vi "GetDough.vi"(8 "error in (no error)":errorcluster, 11 "object in":refnum<class "Pizza(Product).lvclass">) -> (0 "error out":errorcluster, 2 "Dough":string, 3 "object out":refnum<class "Pizza(Product).lvclass">)   [LabVIEW 2014, in "Pizza(Product).lvclass"]
uses:
  Pizza(Product).lvclass
  Pizza(Product).lvclass/Pizza(Product).ctl
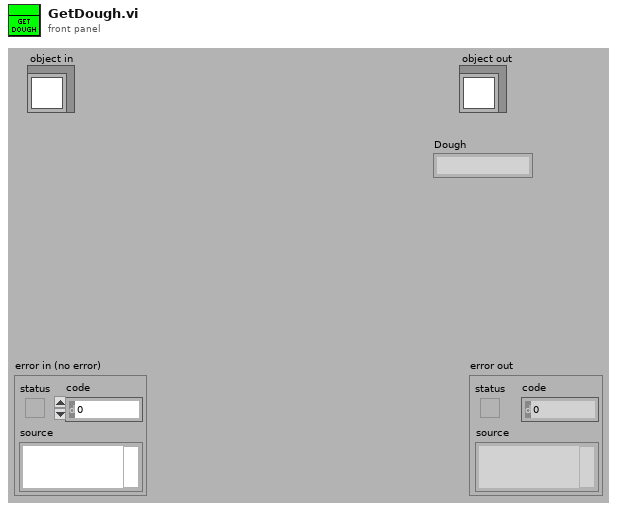
[diagram p1: front panel]
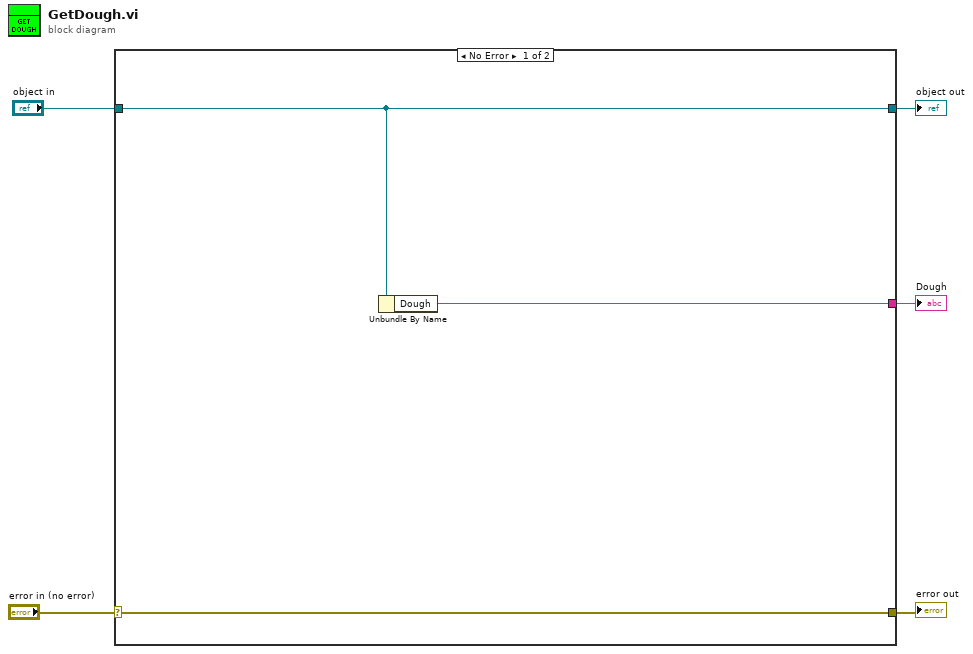
[diagram p0: block diagram]
diagram:
  n1 = case shown="No Error" "error in (no error)" {
    selector: "error in (no error)" -> [w7 w10]
    tunnel: [w7 w10] -> w4
    tunnel: [w6 w9] -> w2
    tunnel: "object in" -> [w6 w9]
    tunnel: [w8 _] -> w1
    frame No Error {
      n2 = Unbundle By Name(w6) -> ("Dough"=w8:string)
    }
    frame Error {
    }
  }
  "error out" <- w4
  "object out" <- w2
  "Dough" <- w1
